vi "VS SLSC Apply Static Properties.vi"(5 "Popup Error?":bool, 7 "Reset?":bool, 8 "error in (no error)":errorcluster, 9 "Configuration Data":T1={"Properties"={"Boolean Properties"=[], "Double Properties"=[], "I32 Properties"=[], "I64 Properties"=[], "String Properties"=[], "U32 Properties"=[], "U64 Properties"=[]}, "Commands"=[], "Reset Commands"=[], "Apply Values on Deployment"=TRUE, "Apply Reset on Undeployment"=TRUE, "Change Commands"=[]}, 10 "SLSC Module Name in":refnum<k21>, 11 "Refnum in":refnum<k21>) -> (0 "error out":errorcluster, 2 "SLSC Module Name out":refnum<k21>, 3 "Refnum out":refnum<k21>)   [LabVIEW 2017, in "SLSC EDS Engine.lvlib"]
uses:
  SLSC EDS Engine.lvlib
  Shared/SLSC Static Settings.ctl
  SLSC CD API/SLSC CD Engine/SLSC Dynamic Channel.ctl
  SLSC CD API/SLSC CD Engine/SLSC Datatype.ctl
  <vilib>/SLSC/Set Generic Property (DBL).vi
  <vilib>/SLSC/Set Generic Property (Bool).vi
  <vilib>/SLSC/Set Generic Property (String).vi
  <vilib>/SLSC/Set Generic Property (I64).vi
  <vilib>/SLSC/Set Generic Property (I32).vi
  <vilib>/SLSC/Set Generic Property (U32).vi
  <vilib>/SLSC/Set Generic Property (U64).vi
  <vilib>/SLSC/Commit Properties for Devices.vi
  <vilib>/SLSC/Execute Command.vi
  <vilib>/SLSC/Execute Device Command.vi
  <vilib>/SLSC/Execute Phys Chan Command.vi
  <vilib>/SLSC/SLSC.lvlib
  SLSC CD API/SLSC CD Shared/SLSC CD Shared.lvlib
  SLSC CD API/SLSC CD Engine/SLSC CD Engine.lvlib
  <vilib>/NI VeriStand/Custom Device Tools/Custom Device Utility Library/Custom Device Utility Library.lvlib
  Shared/SLSC EDS Shared.lvlib
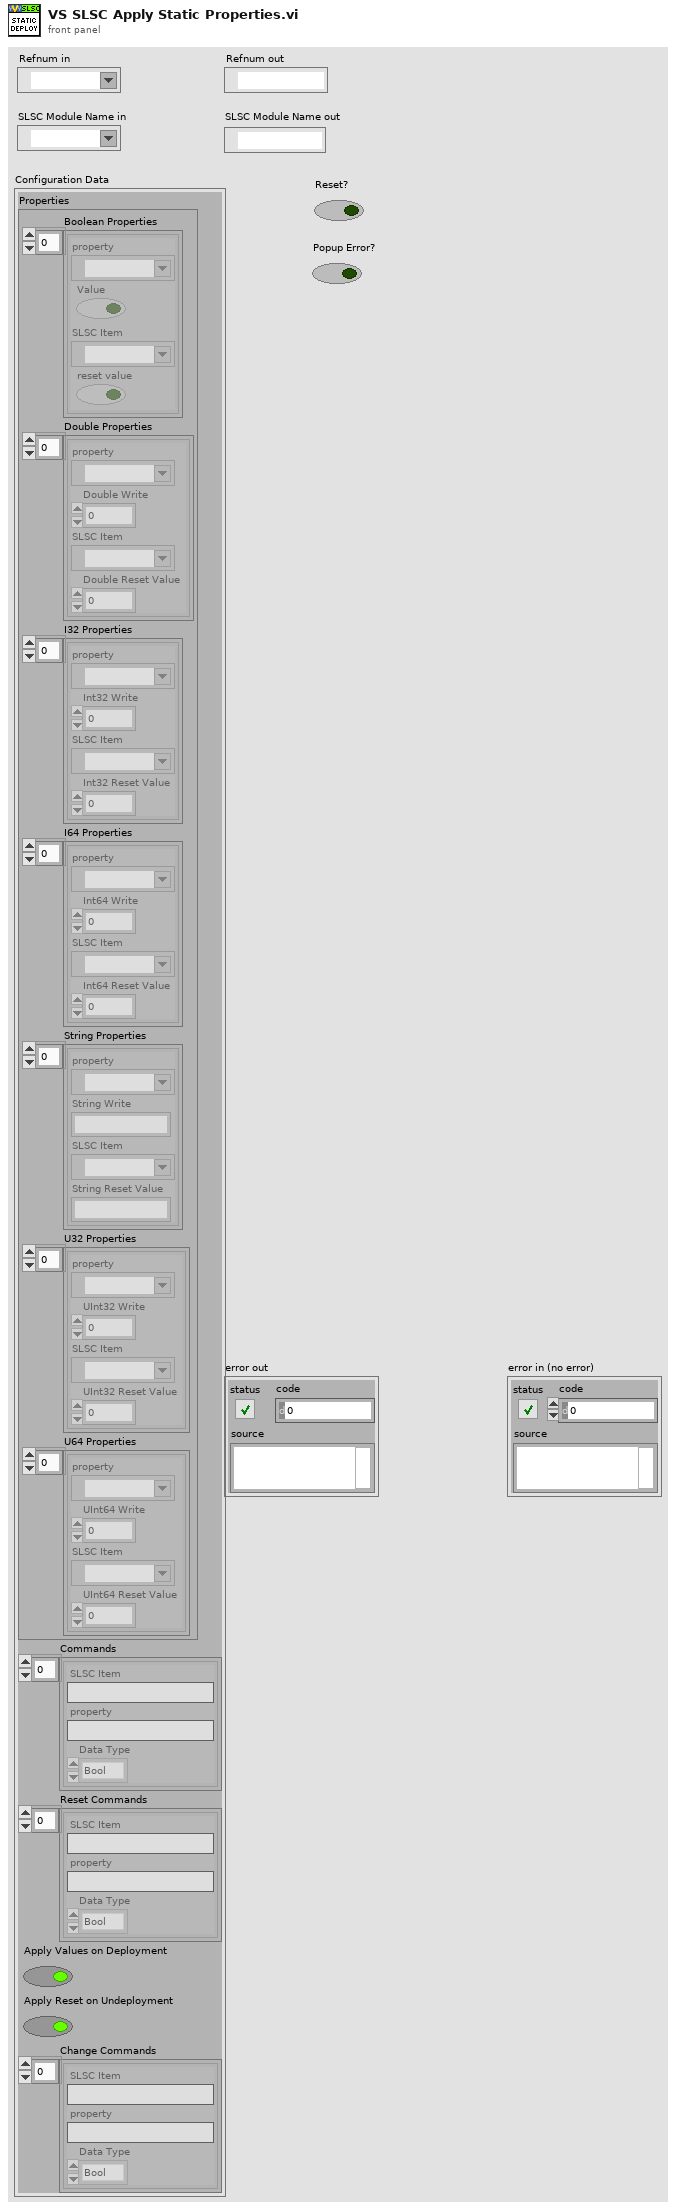
[diagram p1: front panel]
types:
  T1 = typedef "SLSC EDS Shared.lvlib/SLSC Static Settings.ctl" = cluster{"Properties":cluster{"Boolean Properties":cluster{"property":refnum<k21>, "Value":bool, "SLSC Item":refnum<k21>, "reset value":bool}[], "Double Properties":cluster{"property":refnum<k21>, "Double Write":dbl, "SLSC Item":refnum<k21>, "Double Reset Value":dbl}[], "I32 Properties":cluster{"property":refnum<k21>, "Int32 Write":i32, "SLSC Item":refnum<k21>, "Int32 Reset Value":i32}[], "I64 Properties":cluster{"property":refnum<k21>, "Int64 Write":i64, "SLSC Item":refnum<k21>, "Int64 Reset Value":i64}[], "String Properties":cluster{"property":refnum<k21>, "String Write":string, "SLSC Item":refnum<k21>, "String Reset Value":string}[], "U32 Properties":cluster{"property":refnum<k21>, "UInt32 Write":u32, "SLSC Item":refnum<k21>, "UInt32 Reset Value":u32}[], "U64 Properties":cluster{"property":refnum<k21>, "UInt64 Write":u64, "SLSC Item":refnum<k21>, "UInt64 Reset Value":u64}[]}, "Commands":T2[], "Reset Commands":T2[], "Apply Values on Deployment":bool, "Apply Reset on Undeployment":bool, "Change Commands":T2[]}
  T2 = typedef "SLSC CD Shared.lvlib/SLSC Dynamic Channel.ctl" = cluster{"SLSC Item":string, "property":string, "Data Type":T3}
  T3 = typedef "SLSC CD Shared.lvlib/SLSC Datatype.ctl" = enum16{"Bool", "Double", "I32", "I64", "String", "U32", "U64"}
  T4 = cluster{"property":refnum<k21>, "Value":bool, "SLSC Item":refnum<k21>, "reset value":bool}[]
  T5 = cluster{"property":refnum<k21>, "Double Write":dbl, "SLSC Item":refnum<k21>, "Double Reset Value":dbl}[]
  T6 = cluster{"property":refnum<k21>, "Int32 Write":i32, "SLSC Item":refnum<k21>, "Int32 Reset Value":i32}[]
  T7 = cluster{"property":refnum<k21>, "Int64 Write":i64, "SLSC Item":refnum<k21>, "Int64 Reset Value":i64}[]
  T8 = cluster{"property":refnum<k21>, "String Write":string, "SLSC Item":refnum<k21>, "String Reset Value":string}[]
  T9 = cluster{"property":refnum<k21>, "UInt32 Write":u32, "SLSC Item":refnum<k21>, "UInt32 Reset Value":u32}[]
  T10 = cluster{"property":refnum<k21>, "UInt64 Write":u64, "SLSC Item":refnum<k21>, "UInt64 Reset Value":u64}[]
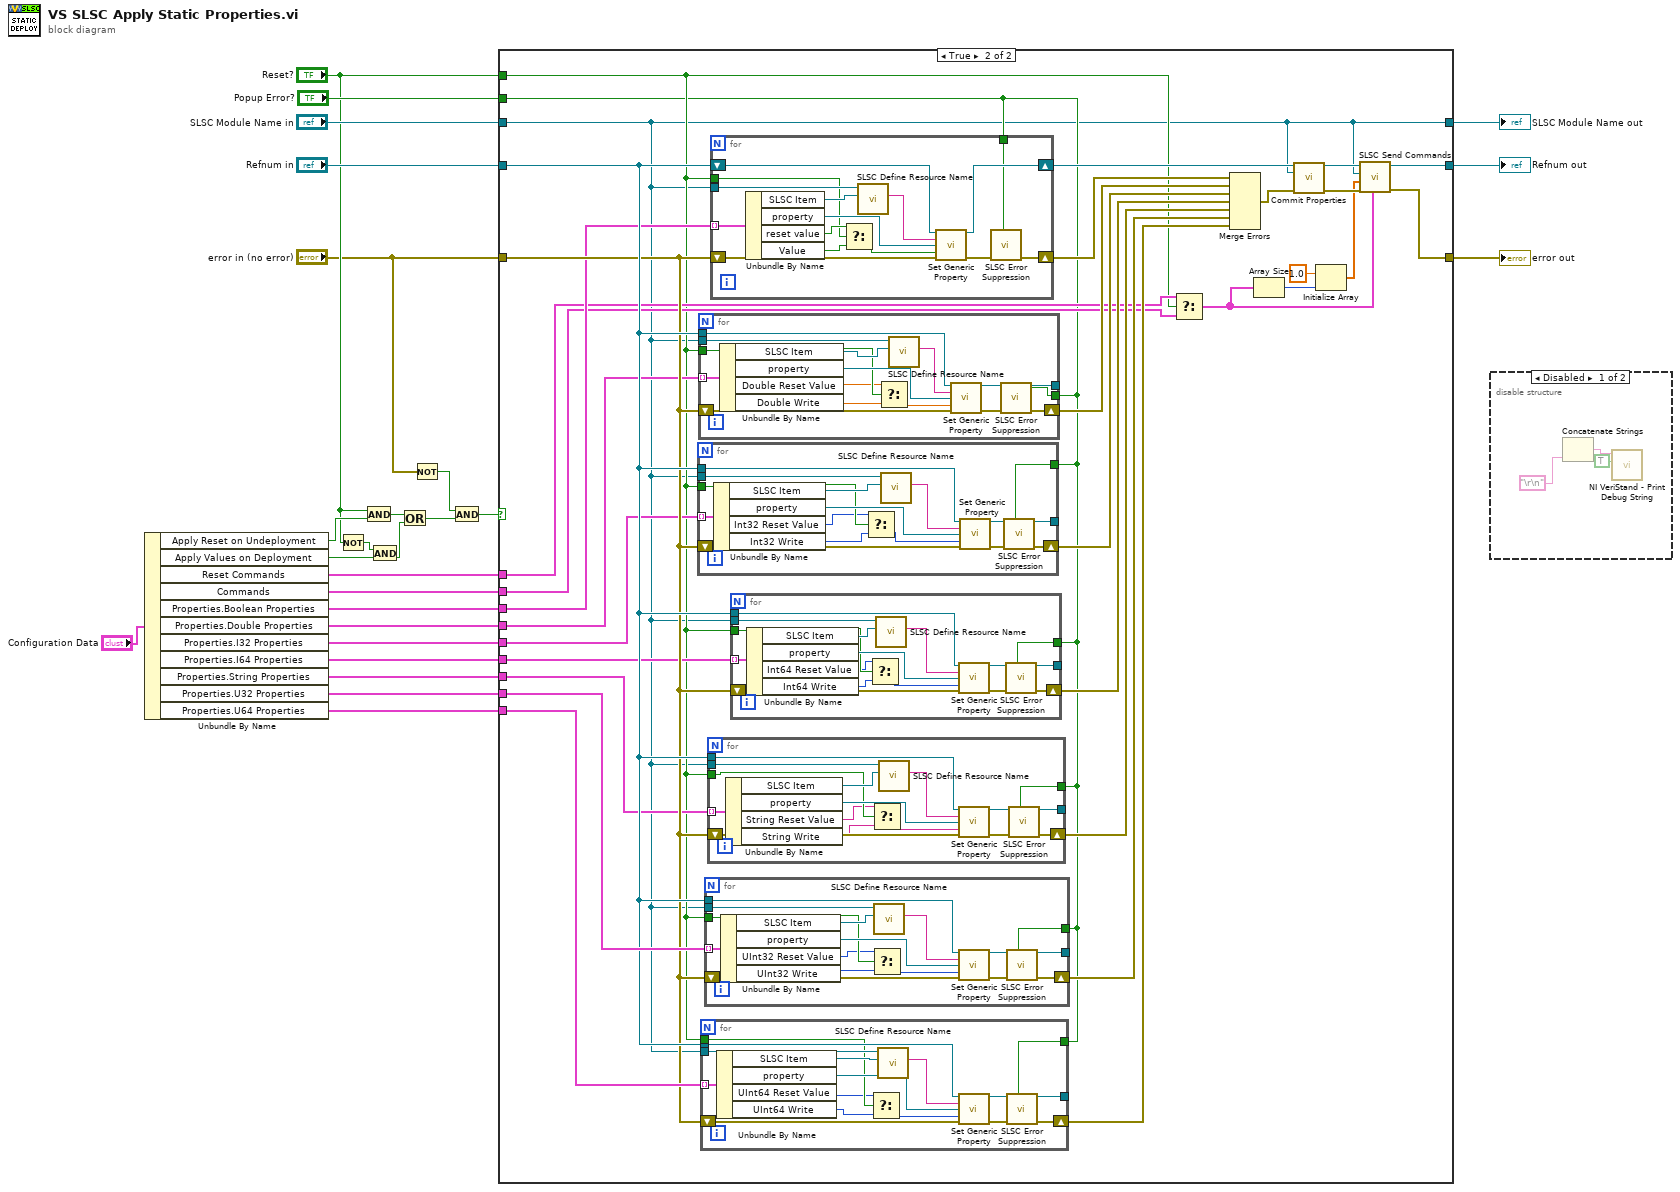
[diagram p0: block diagram]
diagram:
  n1 = Unbundle By Name("Configuration Data") -> ("Apply Reset on Undeployment"=w9:bool, "Apply Values on Deployment"=w7:bool, "Reset Commands"=w13:T2[], "Commands"=w14:T2[], "Properties.Boolean Properties"=w19:T4, "Properties.Double Properties"=w20:T5, "Properties.I32 Properties"=w21:T6, "Properties.I64 Properties"=w22:T7, "Properties.String Properties"=w23:T8, "Properties.U32 Properties"=w25:T9, "Properties.U64 Properties"=w26:T10)
  n2 = Not(x="Reset?") -> (.not. x?=w4:bool)
  n3 = And(x="Reset?", y=w9) -> (x .and. y?=w10:bool)
  n4 = And(x=w4, y=w7) -> (x .and. y?=w6:bool)
  n5 = Or(x=w10, y=w6) -> (x .or. y?=w11:bool)
  n6 = Not(x="error in (no error)") -> (.not. x?=w1:bool)
  n7 = And(x=w1, y=w11) -> (x .and. y?=w3:bool)
  n8 = case shown="True" w3 {
    tunnel: w26 -> [_ w58]
    tunnel: w25 -> [_ w57]
    tunnel: "Refnum in" -> [w29 w56]
    tunnel: "error in (no error)" -> [w27 w55]
    tunnel: w23 -> [_ w53]
    tunnel: w22 -> [_ w50]
    tunnel: w21 -> [_ w49]
    tunnel: w20 -> [_ w47]
    tunnel: w19 -> [_ w45]
    tunnel: [w29 w41] -> w17
    tunnel: "SLSC Module Name in" -> [w28 w30]
    tunnel: [w27 w39] -> w15
    tunnel: w14 -> [_ w34]
    tunnel: w13 -> [_ w33]
    tunnel: "Reset?" -> [_ w32]
    tunnel: "Popup Error?" -> [_ w31]
    tunnel: [w28 w30] -> w12
    frame False {
    }
    frame True {
      n9 = for {
        tunnel: w49 -> [w135] mode=indexing
        tunnel: w56 -> [w131]
        tunnel: [w132] -> _
        shift-right: [w121] -> w51
        shift-left: w55 -> [w133]
        tunnel: w30 -> [w130]
        tunnel: w32 -> [w126]
        tunnel: w31 -> [w122]
        n10 = Unbundle By Name(w135) -> ("SLSC Item"=w129:refnum<k21>, "property"=w134:refnum<k21>, "Int32 Reset Value"=w125:i32, "Int32 Write"=w124:i32)
        n11 = Select(t=w125, s=w126, f=w124) -> (s? t:f=w127:i32)
        n12 = call "SLSC Define Resource Name.vi"("SLSC Item"=w129, "SLSC Module Name"=w130) -> ("Resource"=w128:string)  [unwired: 9 in]
        n13 = call-poly <vilib>:"Set Generic Property.vi"("session in"=w131, "resources"=w128, "property"=w134, "property value"=w127, "error in (no error)"=w133) -> ("session out"=w132:refnum<k21>, "error out"=w123:errorcluster)  [unwired: 9 in]
        n14 = call "SLSC Error Suppression.vi"("error in (no error)"=w123, "Popup Error?"=w122) -> ("error out"=w121:errorcluster)  [unwired: 7 in, 1 out]
      }
      n15 = for {
        tunnel: w47 -> [w150] mode=indexing
        tunnel: w56 -> [w146]
        tunnel: [w147] -> _
        shift-right: [w136] -> w48
        shift-left: w55 -> [w148]
        tunnel: w30 -> [w145]
        tunnel: w32 -> [w141]
        tunnel: w31 -> [w137]
        n16 = Unbundle By Name(w150) -> ("SLSC Item"=w143:refnum<k21>, "property"=w149:refnum<k21>, "Double Reset Value"=w140:dbl, "Double Write"=w139:dbl)
        n17 = Select(t=w140, s=w141, f=w139) -> (s? t:f=w142:dbl)
        n18 = call "SLSC Define Resource Name.vi"("SLSC Item"=w143, "SLSC Module Name"=w145) -> ("Resource"=w144:string)  [unwired: 9 in]
        n19 = call-poly <vilib>:"Set Generic Property.vi"("session in"=w146, "resources"=w144, "property"=w149, "property value"=w142, "error in (no error)"=w148) -> ("session out"=w147:refnum<k21>, "error out"=w138:errorcluster)  [unwired: 9 in]
        n20 = call "SLSC Error Suppression.vi"("error in (no error)"=w138, "Popup Error?"=w137) -> ("error out"=w136:errorcluster)  [unwired: 7 in, 1 out]
      }
      n21 = for {
        tunnel: w58 -> [w75] mode=indexing
        tunnel: w56 -> [w71]
        tunnel: [w72] -> _
        shift-right: [w61] -> w60
        shift-left: w55 -> [w73]
        tunnel: w30 -> [w69]
        tunnel: w32 -> [w66]
        tunnel: w31 -> [w62]
        n22 = Unbundle By Name(w75) -> ("SLSC Item"=w70:refnum<k21>, "property"=w74:refnum<k21>, "UInt64 Reset Value"=w65:u64, "UInt64 Write"=w64:u64)
        n23 = Select(t=w65, s=w66, f=w64) -> (s? t:f=w67:u64)
        n24 = call "SLSC Define Resource Name.vi"("SLSC Item"=w70, "SLSC Module Name"=w69) -> ("Resource"=w68:string)  [unwired: 9 in]
        n25 = call-poly <vilib>:"Set Generic Property.vi"("session in"=w71, "resources"=w68, "property"=w74, "property value"=w67, "error in (no error)"=w73) -> ("session out"=w72:refnum<k21>, "error out"=w63:errorcluster)  [unwired: 9 in]
        n26 = call "SLSC Error Suppression.vi"("error in (no error)"=w63, "Popup Error?"=w62) -> ("error out"=w61:errorcluster)  [unwired: 7 in, 1 out]
      }
      n27 = for {
        tunnel: w57 -> [w90] mode=indexing
        tunnel: w56 -> [w86]
        tunnel: [w87] -> _
        shift-right: [w76] -> w59
        shift-left: w55 -> [w88]
        tunnel: w30 -> [w85]
        tunnel: w32 -> [w81]
        tunnel: w31 -> [w77]
        n28 = Unbundle By Name(w90) -> ("SLSC Item"=w84:refnum<k21>, "property"=w89:refnum<k21>, "UInt32 Reset Value"=w80:u32, "UInt32 Write"=w79:u32)
        n29 = Select(t=w80, s=w81, f=w79) -> (s? t:f=w82:u32)
        n30 = call "SLSC Define Resource Name.vi"("SLSC Item"=w84, "SLSC Module Name"=w85) -> ("Resource"=w83:string)  [unwired: 9 in]
        n31 = call-poly <vilib>:"Set Generic Property.vi"("session in"=w86, "resources"=w83, "property"=w89, "property value"=w82, "error in (no error)"=w88) -> ("session out"=w87:refnum<k21>, "error out"=w78:errorcluster)  [unwired: 9 in]
        n32 = call "SLSC Error Suppression.vi"("error in (no error)"=w78, "Popup Error?"=w77) -> ("error out"=w76:errorcluster)  [unwired: 7 in, 1 out]
      }
      n33 = for {
        tunnel: w53 -> [w105] mode=indexing
        tunnel: w56 -> [w101]
        tunnel: [w102] -> _
        shift-right: [w91] -> w54
        shift-left: w55 -> [w103]
        tunnel: w30 -> [w100]
        tunnel: w32 -> [w96]
        tunnel: w31 -> [w92]
        n34 = Unbundle By Name(w105) -> ("SLSC Item"=w99:refnum<k21>, "property"=w104:refnum<k21>, "String Reset Value"=w95:string, "String Write"=w94:string)
        n35 = Select(t=w95, s=w96, f=w94) -> (s? t:f=w97:string)
        n36 = call "SLSC Define Resource Name.vi"("SLSC Item"=w99, "SLSC Module Name"=w100) -> ("Resource"=w98:string)  [unwired: 9 in]
        n37 = call-poly <vilib>:"Set Generic Property.vi"("session in"=w101, "resources"=w98, "property"=w104, "property value"=w97, "error in (no error)"=w103) -> ("session out"=w102:refnum<k21>, "error out"=w93:errorcluster)  [unwired: 9 in]
        n38 = call "SLSC Error Suppression.vi"("error in (no error)"=w93, "Popup Error?"=w92) -> ("error out"=w91:errorcluster)  [unwired: 7 in, 1 out]
      }
      n39 = for {
        tunnel: w45 -> [w165] mode=indexing
        shift-right: [w151] -> w46
        shift-left: w55 -> [w163]
        tunnel: w30 -> [w160]
        shift-right: [w162] -> w43
        shift-left: w56 -> [w161]
        tunnel: w32 -> [w155]
        tunnel: w31 -> [w152]
        n40 = Unbundle By Name(w165) -> ("SLSC Item"=w159:refnum<k21>, "property"=w164:refnum<k21>, "reset value"=w156:bool, "Value"=w154:bool)
        n41 = Select(t=w156, s=w155, f=w154) -> (s? t:f=w157:bool)
        n42 = call "SLSC Define Resource Name.vi"("SLSC Item"=w159, "SLSC Module Name"=w160) -> ("Resource"=w158:string)  [unwired: 9 in]
        n43 = call-poly <vilib>:"Set Generic Property.vi"("session in"=w161, "resources"=w158, "property"=w164, "property value"=w157, "error in (no error)"=w163) -> ("session out"=w162:refnum<k21>, "error out"=w153:errorcluster)  [unwired: 9 in]
        n44 = call "SLSC Error Suppression.vi"("error in (no error)"=w153, "Popup Error?"=w152) -> ("error out"=w151:errorcluster)  [unwired: 7 in, 1 out]
      }
      n45 = for {
        tunnel: w50 -> [w120] mode=indexing
        tunnel: w56 -> [w116]
        tunnel: [w117] -> _
        shift-right: [w106] -> w52
        shift-left: w55 -> [w118]
        tunnel: w30 -> [w114]
        tunnel: w32 -> [w111]
        tunnel: w31 -> [w107]
        n46 = Unbundle By Name(w120) -> ("SLSC Item"=w113:refnum<k21>, "property"=w119:refnum<k21>, "Int64 Reset Value"=w110:i64, "Int64 Write"=w109:i64)
        n47 = Select(t=w110, s=w111, f=w109) -> (s? t:f=w112:i64)
        n48 = call "SLSC Define Resource Name.vi"("SLSC Item"=w113, "SLSC Module Name"=w114) -> ("Resource"=w115:string)  [unwired: 9 in]
        n49 = call-poly <vilib>:"Set Generic Property.vi"("session in"=w116, "resources"=w115, "property"=w119, "property value"=w112, "error in (no error)"=w118) -> ("session out"=w117:refnum<k21>, "error out"=w108:errorcluster)  [unwired: 9 in]
        n50 = call "SLSC Error Suppression.vi"("error in (no error)"=w108, "Popup Error?"=w107) -> ("error out"=w106:errorcluster)  [unwired: 7 in, 1 out]
      }
      n51 = Select(t=w33, s=w32, f=w34) -> (s? t:f=w35:T2[])
      n52 = Merge Errors(w46, w48, w51, w52, w54, w59, w60) -> (w44:errorcluster)
      n53 = Array Size(array=w35) -> (size(s)=w38:i32)
      n54 = call-poly <vilib>:"Commit Properties.vi"("session in"=w43, "devices"=w30, "error in (no error)"=w44) -> ("session out"=w42:refnum<k21>, "error out"=w40:errorcluster)  [unwired: 11 in]
      n55 = Initialize Array(1.0 ("element"), w38) -> (w36:dbl[])
      n56 = call "SLSC Send Commands.vi"("SLSC Dynamic Commands"=w35, "error in"=w40, "Values"=w36, "SLSC Module Name"=w30, "session in"=w42) -> ("error out"=w39:errorcluster, "session out"=w41:refnum<k21>)  [unwired: 4 in, 1 out]
    }
  }
  "SLSC Module Name out" <- w12
  "error out" <- w15
  "Refnum out" <- w17
  n57 = disable-structure shown="Disabled" {
    frame Disabled {
      n58 = Concatenate Strings("\r\n") -> (w167:string)  [unwired: 2 in]
      n59 = call <vilib>:"NI VeriStand - Print Debug String.vi"("Add to log file? (T)"=TRUE, "Message"=w167) -> ()  [unwired: 9 in, 1 out]
    }
    frame Enabled {
    }
  }
